vi "Main.vi"() -> ()   [LabVIEW 2016]
doc: "The myRIO Project template acquires acceleration data from the onboard accelerometer and displays the changes of acceleration values in a waveform chart."
panel:
  out "path":bool[][](array[boolean])
  in  "USE MANUAL ROADBLOCKS":bool
  out "raw string data":string
  out "roadblock names":string[](array[string])
  in  "pickupLocations":bool[](array[boolean])=[TRUE, TRUE, FALSE]
  in  "pause":bool
  in  "go":bool
  out "speed":dbl=0.11
  in  "overwrite angle":bool
  in  "Source":u16(ring) items=["Odometry", "Lidar"]
  in  "Max. Speed":dbl=0.11
  out "rotated coordinate system":cluster{"Line":cluster{"X":dbl, "Y":dbl}[]}[](graph)=[{"Line"=[{"X"=28.576616461317627, "Y"=357.36358956169147}, {"X"=-4.74077116119355, "Y"=343.61280769162283}, {"X"=-7.350479867352021, "Y"=344.4851372177861}, {"X"=-8.138056777246447, "Y"=346.20981930296045}, {"X"=-7.0881796754405855, "Y"=348.7533004615932}, {"X"=-8.765481040597024, "Y"=350.0749055793108}, {"X"=-8.600379041051553, "Y"=352.2039244346708}, {"X"=-8.419805687206917, "Y"=354.32624780014754}, {"X"=-8.223837019347911, "Y"=356.44176618363844}, {"X"=-8.938032992413582, "Y"=358.1715820073938}, {"X"=-9.64160157058302, "Y"=359.9057474919626}, {"X"=-11.264578053362584, "Y"=361.2767942037909}, {"X"=-11.949049611130476, "Y"=363.0251766457427}, {"X"=-12.622780410928328, "Y"=364.77772601341337}, {"X"=-13.285745087172302, "Y"=366.53437632430945}, {"X"=-8.305129505171124, "Y"=370.3618672176699}, {"X"=-8.933911813679401, "Y"=372.091919800773}, {"X"=-9.552066882451356, "Y"=373.82579795183943}, {"X"=-8.269612100595452, "Y"=376.2176945222226}, {"X"=-8.862464396842654, "Y"=377.94741894033393}, {"X"=-10.393615033779838, "Y"=379.3652403911355}, {"X"=-10.016273419447543, "Y"=381.41761785287076}, {"X"=-10.577186705547717, "Y"=383.15796169626856}, {"X"=-8.263702090581091, "Y"=385.7956786540522}, {"X"=-8.797785092278218, "Y"=387.52518650617935}, {"X"=-9.321245979333298, "Y"=389.25793887250137}, {"X"=-9.834065043739827, "Y"=390.99387051587115}, {"X"=-13.22100825471199, "Y"=391.9095000800054}, {"X"=-13.717484233486346, "Y"=393.6693102999656}, {"X"=-10.343589355728568, "Y"=396.4827380376795}, {"X"=-10.81205864051907, "Y"=398.22480665727596}, {"X"=-11.269829974406946, "Y"=399.96971695641616}, {"X"=-9.777762208684806, "Y"=402.2070954360229}, {"X"=-9.240072095703283, "Y"=404.18447681452164}, {"X"=-9.661305173161736, "Y"=405.91962939644634}, {"X"=-10.071883624935197, "Y"=407.6573339521877}, {"X"=-10.471791992977046, "Y"=409.39752505815153}, {"X"=-10.861015220963111, "Y"=411.1401371971261}, {"X"=-11.239538654859018, "Y"=412.8851047607493}, {"X"=-14.54489110801353, "Y"=414.0233951038116}, {"X"=-8.042797116220015, "Y"=417.16975136641827}, {"X"=-8.384376585253563, "Y"=418.89731316305176}, {"X"=-8.715349504241715, "Y"=420.6269383310432}, {"X"=-9.035703412241162, "Y"=422.3585617509825}, {"X"=-9.34542624810831, "Y"=424.0921182282268}, {"X"=-9.644506350953407, "Y"=425.8275424953543}, {"X"=-9.93293246057965, "Y"=427.5647692146224}, {"X"=-11.198655470293886, "Y"=429.14903464229513}, {"X"=-11.466672030825464, "Y"=430.89573491513625}, {"X"=-11.723965994630248, "Y"=432.64404682553766}, {"X"=-18.905020724190877, "Y"=433.43849566056014}, {"X"=-14.189269156327327, "Y"=435.8844303075074}, {"X"=-9.454690928780451, "Y"=438.2709538865383}, {"X"=-9.666769274690068, "Y"=440.0067816765684}, {"X"=-9.868192789194438, "Y"=441.7438780783978}, {"X"=-10.058953888811914, "Y"=443.4821776913292}, {"X"=-7.254062500877922, "Y"=445.5214102373096}, {"X"=-7.421694309173745, "Y"=447.24359873735864}, {"X"=-4.590318737091252, "Y"=449.22992564923106}, {"X"=-7.725241095683145, "Y"=450.6908993097107}, {"X"=-9.855438786401749, "Y"=452.2649151077689}, {"X"=-9.981644256507991, "Y"=454.00293840806137}, {"X"=-10.097183040343793, "Y"=455.74170337276314}, {"X"=-10.2020507879393, "Y"=457.48114453835586}, {"X"=-10.296243551082966, "Y"=459.221196415863}, {"X"=-10.379757783470552, "Y"=460.96179349331453}, {"X"=-12.451089774345235, "Y"=462.62541047915863}, {"X"=-12.51367557754827, "Y"=464.3791653611051}, {"X"=-12.565499364932691, "Y"=466.13327124838077}, {"X"=-12.606559185362244, "Y"=467.8876620998903}, {"X"=-11.636954252712883, "Y"=469.6564672629717}, {"X"=-11.656413628399832, "Y"=471.4050943456118}, {"X"=-7.665150667473995, "Y"=473.1615040251902}, {"X"=-6.663187179987403, "Y"=474.8814827168105}, {"X"=-6.650680093319181, "Y"=476.5994929789812}, {"X"=-6.627631729298514, "Y"=478.31739415805316}, {"X"=-6.594042955683392, "Y"=480.03512157601784}, {"X"=-6.5499150370721395, "Y"=481.752610561409}, {"X"=-6.495249634855895, "Y"=483.4697964517369}, {"X"=-6.430048807156254, "Y"=485.1866145959235}, {"X"=-7.3532030238397965, "Y"=486.95014622935224}, {"X"=-7.266631020635884, "Y"=488.67216315996683}, {"X"=-8.167728798156418, "Y"=490.45301669341313}, {"X"=-8.059648252626573, "Y"=492.17996551967616}, {"X"=-5.946113080761734, "Y"=493.7629274424393}, {"X"=-5.817765125964911, "Y"=495.47618238279114}, {"X"=-5.678907252593433, "Y"=497.18861754335745}, {"X"=-4.533602281761773, "Y"=498.8101755503944}, {"X"=-4.374311584895565, "Y"=500.5146684743988}, {"X"=-4.204565314664592, "Y"=502.21815192246373}, {"X"=-9.98907306792114, "Y"=504.57041994725495}, {"X"=-1.8468641884958856, "Y"=505.3930189953423}, {"X"=-9.588938254255936, "Y"=508.0449096021341}, {"X"=-10.364844281303931, "Y"=509.9068374384244}, {"X"=-9.14619623718312, "Y"=511.514227364647}, {"X"=-7.918541104854057, "Y"=513.1080304041075}, {"X"=-8.660913692021893, "Y"=514.9778507683}, {"X"=-7.4137925848477835, "Y"=516.5564685803645}, {"X"=-7.145558462231008, "Y"=518.2782999508851}, {"X"=-7.853387999552297, "Y"=520.1614681851706}, {"X"=-9.534235248411392, "Y"=522.224060739526}, {"X"=-9.231185517333586, "Y"=523.9587962108145}, {"X"=-10.884409037757564, "Y"=526.0539356004363}, {"X"=-10.557834219672543, "Y"=527.7968834860404}, {"X"=-8.258253373376306, "Y"=529.1513889314982}, {"X"=-4.972857724789094, "Y"=530.2805060927069}, {"X"=-9.514030681444524, "Y"=533.0132452292144}, {"X"=-8.16734377467003, "Y"=534.5364235287593}, {"X"=-7.788772537104705, "Y"=536.2625401348871}, {"X"=-7.399617173649688, "Y"=537.9863013779125}, {"X"=-6.9998923357846365, "Y"=539.7076423591985}, {"X"=-6.589613072923612, "Y"=541.4264982712307}, {"X"=-6.16879483184897, "Y"=543.1428044000553}, {"X"=-5.737453456129742, "Y"=544.8564961277164}, {"X"=-6.263070235534087, "Y"=546.8205136322952}, {"X"=-5.809161085484845, "Y"=548.5347145911218}, {"X"=-5.344742340798291, "Y"=550.2460981464135}, {"X"=-2.9445431772094253, "Y"=551.4130604618009}, {"X"=-2.462517159902575, "Y"=553.106812867996}, {"X"=-1.9701075472106027, "Y"=554.797575733741}, {"X"=-14.872292004672545, "Y"=560.5234868358712}, {"X"=-15.289850128660532, "Y"=562.5845676530818}, {"X"=-14.739044634956315, "Y"=564.3538591382237}, {"X"=-14.177393341546122, "Y"=566.1197376379802}, {"X"=-13.604917394283916, "Y"=567.8821366680233}, {"X"=-13.021638346565624, "Y"=569.6409898750259}, {"X"=-12.42757815851752, "Y"=571.3962310391589}, {"X"=-9.934301657009087, "Y"=572.4892136921314}, {"X"=-13.091585246825389, "Y"=575.565768386433}, {"X"=-8.700702889770241, "Y"=575.9579170572881}, {"X"=-9.005971749992511, "Y"=578.0331411139174}, {"X"=-8.360493883773245, "Y"=579.7635846311488}, {"X"=-7.704410366678644, "Y"=581.4900349955396}, {"X"=-7.037745899882566, "Y"=583.2124272072089}, {"X"=-11.006619516480896, "Y"=586.7783465917362}, {"X"=-11.234378317351457, "Y"=588.8961258843899}, {"X"=-10.52220448051105, "Y"=590.6400381546518}, {"X"=-9.79934360561333, "Y"=592.379547779745}, {"X"=-9.06582290796166, "Y"=594.1145892681152}, {"X"=-8.321670004195653, "Y"=595.8450972964314}, {"X"=-7.56691291125162, "Y"=597.571006712044}, {"X"=-7.714074863751819, "Y"=599.7013407976909}, {"X"=-6.02570022071302, "Y"=601.0087699626846}, {"X"=-7.96152054987607, "Y"=603.9812598891432}, {"X"=-7.1568476814880455, "Y"=605.7048063082864}, {"X"=-6.341614478824056, "Y"=607.4233829022542}, {"X"=-5.515851634953492, "Y"=609.1369249676097}, {"X"=-4.679590239380502, "Y"=610.8453679904626}, {"X"=-4.726949489757828, "Y"=612.9965395573656}, {"X"=-11.888924814779273, "Y"=618.7803947764087}, {"X"=-10.993372229540284, "Y"=620.5277607055597}, {"X"=-10.08711486704459, "Y"=622.2695987336806}, {"X"=-10.053013460071043, "Y"=624.4755423042335}, {"X"=-5.60283876818562, "Y"=624.3111076715884}, {"X"=-4.673468700387673, "Y"=626.0197987877557}, {"X"=-8.103788909902335, "Y"=630.1521022214033}, {"X"=-7.138532093630772, "Y"=631.8760289240817}, {"X"=-5.294712387779498, "Y"=633.0974419467224}, {"X"=-5.176376265912438, "Y"=635.3059521780373}, {"X"=-6.765084175222, "Y"=638.5333381993366}, {"X"=-5.748426262510748, "Y"=640.2488929897848}, {"X"=-7.287928028799342, "Y"=643.5113098946317}, {"X"=-7.9454418991443845, "Y"=646.2758804458762}, {"X"=-8.579530684886436, "Y"=649.0548736967197}, {"X"=-11.727686448201723, "Y"=653.4482191933557}, {"X"=-10.61941912656988, "Y"=655.193943170491}, {"X"=-9.500461106804153, "Y"=656.9328340844199}, {"X"=-8.370854517041835, "Y"=658.6648264668819}, {"X"=-3.9004938613651916, "Y"=658.1739773753948}, {"X"=-2.7633771773371905, "Y"=659.8715856406279}, {"X"=-1.615865570714334, "Y"=661.5621847320599}, {"X"=0.36419694891867493, "Y"=662.6765111347985}, {"X"=-3.383286648068747, "Y"=667.7932714052793}, {"X"=-5.447766123981808, "Y"=671.8045116821027}, {"X"=-5.850150506567218, "Y"=674.6798321014182}, {"X"=-4.611719100169125, "Y"=676.3890925168814}, {"X"=-6.580231930976424, "Y"=680.4673331146699}, {"X"=-6.907658127202353, "Y"=683.379118347888}, {"X"=-5.615828996583957, "Y"=685.0947037465218}, {"X"=-9.073174580468503, "Y"=690.4554761805456}, {"X"=-7.737884969217532, "Y"=692.184215727906}, {"X"=-7.177761300675797, "Y"=694.523276104051}, {"X"=-6.599485849851021, "Y"=696.86366520989}, {"X"=-6.78111983557892, "Y"=699.8333904921269}, {"X"=-5.3883315711452155, "Y"=701.5478897193765}, {"X"=-2.444386340660799, "Y"=701.9785237132016}, {"X"=-1.0385174240079778, "Y"=703.6663728624455}, {"X"=-3.434562208301088, "Y"=708.580807116901}, {"X"=-1.9881638024811537, "Y"=710.274607584932}, {"X"=-2.04030174789159, "Y"=713.2722138796564}, {"X"=-3.566781716796527, "Y"=717.601263778914}, {"X"=-3.5577118068576965, "Y"=720.6268360737213}, {"X"=-13.171025825242452, "Y"=732.3731469219651}, {"X"=-12.316573107347551, "Y"=734.8009151196794}, {"X"=-10.709123941989048, "Y"=736.5487209959161}, {"X"=-8.36119953858173, "Y"=737.602950034046}, {"X"=-7.462204307042384, "Y"=740.014579243237}, {"X"=-6.544192478265359, "Y"=742.4250859977826}, {"X"=-5.607144139577372, "Y"=744.8343275597374}, {"X"=-6.78938941218064, "Y"=749.3463147892161}, {"X"=-5.801261365891946, "Y"=751.7656776696217}, {"X"=-3.3857187638355413, "Y"=752.7631082289083}, {"X"=-1.6682237743222572, "Y"=754.4557772798655}, {"X"=-2.721797020952863, "Y"=759.0125399333904}, {"X"=-9.257161622796275, "Y"=769.376046154616}, {"X"=-8.124105020179286, "Y"=771.8315738894411}, {"X"=-6.2895189261544715, "Y"=773.5529581734131}, {"X"=-6.476932476945194, "Y"=777.469596394551}, {"X"=-4.60778313473719, "Y"=779.1807676836203}, {"X"=-9.412491430211844, "Y"=788.3181686710523}, {"X"=-10.796000795056557, "Y"=793.786450495438}, {"X"=-9.48590644158304, "Y"=796.2757356954651}, {"X"=-9.465193730872045, "Y"=800.2728678468713}, {"X"=-7.456069892235803, "Y"=802.0019454971552}, {"X"=-9.953492337332364, "Y"=809.0661525397925}, {"X"=-10.452816880429737, "Y"=813.8695496847113}, {"X"=-14.71904081923617, "Y"=823.3223156412832}, {"X"=-14.461784812557255, "Y"=827.4102231493271}, {"X"=-12.286055232686806, "Y"=829.1694484530829}, {"X"=-10.099572206775065, "Y"=830.9152906141896}, {"X"=-7.90241805467241, "Y"=832.6476839026767}, {"X"=-8.142298346368534, "Y"=837.5302859639576}, {"X"=-10.76092125893905, "Y"=845.6079084090223}, {"X"=-8.473602449144096, "Y"=847.3440830746283}, {"X"=-6.175673730000483, "Y"=849.0661903328643}, {"X"=-3.867221617225141, "Y"=850.7741653473654}, {"X"=-14.4701675724736, "Y"=870.2731731543768}, {"X"=-12.031435717846477, "Y"=872.0316430108596}, {"X"=-10.736720367624855, "Y"=875.4080668442864}, {"X"=-8.266551678719338, "Y"=877.1435320364542}, {"X"=-9.18968465743086, "Y"=883.8048036432882}, {"X"=-6.668023682607554, "Y"=885.5306183365925}, {"X"=-5.807327705133503, "Y"=889.732125342123}, {"X"=-9.874120088076722, "Y"=901.4427014978764}, {"X"=-9.43196911126148, "Y"=906.5210795125762}, {"X"=-6.770919127109551, "Y"=908.247953207868}, {"X"=-7.8556784022915735, "Y"=915.8652250552609}, {"X"=-7.794495750848455, "Y"=921.8177480003112}, {"X"=-8.196978458223043, "Y"=928.6363521433555}, {"X"=-13.736242524766965, "Y"=944.01214617937}, {"X"=-12.90807900096081, "Y"=949.191676137402}, {"X"=-10.49562725444406, "Y"=951.7989619216245}, {"X"=-9.072336663828139, "Y"=956.1205170615633}, {"X"=-10.106116753702281, "Y"=964.7729386898258}, {"X"=-12.033340910816094, "Y"=975.1942226072335}, {"X"=-9.440100589363794, "Y"=977.8079205692866}, {"X"=-6.34164261841255, "Y"=979.5335022037527}, {"X"=-7.539061333916038, "Y"=989.1428785911435}, {"X"=-5.317274566394929, "Y"=992.6186075930843}, {"X"=-4.466407579703116, "Y"=998.7381077790387}, {"X"=-3.0886008324087584, "Y"=1003.9797849534243}, {"X"=-9.422390748874534, "Y"=1024.34690294733}, {"X"=-7.3923625430387006, "Y"=1028.7485725817364}, {"X"=-7.993983839324244, "Y"=1038.5166213778946}, {"X"=-4.963396007688061, "Y"=1041.130015874826}, {"X"=-9.73820276004102, "Y"=1059.936700929226}, {"X"=-6.994393661101242, "Y"=1063.4688956165824}, {"X"=-4.217863479354435, "Y"=1066.9894223036495}, {"X"=-8.099501387073303, "Y"=1085.03185348001}, {"X"=-5.580944645459169, "Y"=1089.479932503771}, {"X"=-3.0183513268182196, "Y"=1093.920017711641}, {"X"=-4.826984283811328, "Y"=1108.4267291040496}, {"X"=-2.1144303473452055, "Y"=1112.8766086225169}, {"X"=-7.5501607217547075, "Y"=1136.653061681427}, {"X"=-3.4770828654445154, "Y"=1138.3640566479803}, {"X"=-2.802682121336943, "Y"=1148.3793758627119}, {"X"=-5.373595942088059, "Y"=1166.7612389698077}, {"X"=-5.892059617806865, "Y"=1180.5491152580664}, {"X"=-2.6347402787606597, "Y"=1185.046005847571}, {"X"=-3.6042542742794126, "Y"=1200.74343475171}, {"X"=-5.4419866034307915, "Y"=1219.2890159791455}, {"X"=-7.062321077849106, "Y"=1237.8838873573395}, {"X"=-4.739017247575703, "Y"=1246.1762423118103}, {"X"=-1.3256554817880328, "Y"=1251.6397452980111}, {"X"=-3.0897310820254233, "Y"=1272.2099762036185}, {"X"=-2.362195675266321, "Y"=1286.201649046942}, {"X"=-3.3662561011780667, "Y"=1305.9075309674656}, {"X"=-2.2805666636053274, "Y"=1319.9506001401144}, {"X"=-0.42513081455462043, "Y"=1332.105766246754}, {"X"=2.1651956347232613, "Y"=1342.3604898886258}, {"X"=-2.724098560849768, "Y"=1377.4813018627735}, {"X"=1.109073246825858, "Y"=1384.907078098183}, {"X"=-1.1450318426243484, "Y"=1413.4372678254877}, {"X"=-0.8631985957002826, "Y"=1434.3356531193622}, {"X"=0.7392338813229458, "Y"=1451.4121917703867}, {"X"=2.2784130196424144, "Y"=1469.469543667663}, {"X"=1.9752874456671066, "Y"=1495.2760742742785}, {"X"=1.72809958998522, "Y"=1522.0909465154327}, {"X"=2.0448527388076627, "Y"=1547.9768043111544}, {"X"=2.669275799484467, "Y"=1573.8973336442273}, {"X"=1.2725041271489772, "Y"=1609.5746679412048}, {"X"=1.665421931336084, "Y"=1639.4658562714153}, {"X"=1.9732061027862642, "Y"=1671.3444819554675}, {"X"=3.522186165777555, "Y"=1699.3556174324276}, {"X"=4.7779344628372655, "Y"=1730.325593190843}, {"X"=4.982894058226975, "Y"=1768.1794664657875}, {"X"=7.612329623712583, "Y"=1796.272690601469}, {"X"=7.330335818030846, "Y"=1841.068557357675}, {"X"=7.03358539097519, "Y"=1888.864307100026}, {"X"=8.029275882144532, "Y"=1932.7779692274896}, {"X"=6.4426973114146335, "Y"=1994.4601436141454}, {"X"=10.107360058679774, "Y"=2029.5927571615584}, {"X"=13.228782674090837, "Y"=2070.6583560051076}, {"X"=-9.24412840866512, "Y"=2977.808666395851}, {"X"=6.126099747780017, "Y"=2979.4953961187844}]}, {"Line"=[{"X"=68.62973356513766, "Y"=4051.851402285283}, {"X"=90.94562316458712, "Y"=4046.0491940237675}, {"X"=112.9134263637961, "Y"=4046.102068397886}, {"X"=135.1073891816279, "Y"=4040.0243951170473}, {"X"=156.99253314549912, "Y"=4040.8054046682064}, {"X"=178.88205731223576, "Y"=4041.4521147981895}, {"X"=200.75480715528755, "Y"=4042.964294474817}, {"X"=222.58577721259627, "Y"=4048.341939900227}, {"X"=244.52030991588802, "Y"=4048.586035577704}, {"X"=266.45592745072076, "Y"=4048.6955388976476}, {"X"=288.3918039534931, "Y"=4048.670445737322}, {"X"=310.32711355085127, "Y"=4048.5107570414684}, {"X"=332.2610303907877, "Y"=4048.2164788222763}, {"X"=354.19272867373047, "Y"=4047.7876221591546}, {"X"=376.1213826836351, "Y"=4047.2242031983146}, {"X"=398.1508201093675, "Y"=4049.524417211289}, {"X"=420.17133524166366, "Y"=4050.689560763215}, {"X"=442.11655318347863, "Y"=4049.7212500549867}, {"X"=464.10869061670405, "Y"=4049.616884178716}, {"X"=486.0464996304325, "Y"=4048.3789991189515}, {"X"=507.97630015117113, "Y"=4047.006529496461}, {"X"=530.2554945953639, "Y"=4050.4866777392676}, {"X"=552.5084528865657, "Y"=4052.8307942088063}, {"X"=574.4643179809686, "Y"=4051.0504379037943}, {"X"=596.4088457014934, "Y"=4049.135396457895}, {"X"=618.3412098490757, "Y"=4047.0857419713357}, {"X"=640.2605846826016, "Y"=4044.9015516124505}, {"X"=662.4910740439232, "Y"=4045.565259217772}, {"X"=684.4002882619448, "Y"=4043.1101990075686}, {"X"=706.7760296379319, "Y"=4044.4916054787773}, {"X"=728.6778223886847, "Y"=4041.7648381005847}, {"X"=752.5525807322003, "Y"=4053.771131255632}, {"X"=776.3142398765136, "Y"=4063.637560662127}, {"X"=798.4770279617144, "Y"=4061.47321142267}, {"X"=821.6884553762941, "Y"=4066.091855419856}, {"X"=844.8193293479787, "Y"=4069.572828702131}, {"X"=867.3614643563512, "Y"=4068.958442120934}, {"X"=890.9319526498374, "Y"=4074.116323245808}, {"X"=913.0120525683635, "Y"=4070.259038689616}, {"X"=935.2492170083682, "Y"=4067.2498016412865}, {"X"=958.9709613722258, "Y"=4071.9616531487213}, {"X"=981.2297625705849, "Y"=4068.6680884687785}, {"X"=1004.470050173194, "Y"=4070.1365788299113}, {"X"=1028.986337704895, "Y"=4077.3272810986987}, {"X"=1051.5060010466395, "Y"=4074.5777230442354}, {"X"=1074.454803523784, "Y"=4073.639653488076}, {"X"=1097.6445680760262, "Y"=4073.530156097562}]}, {"Line"=[{"X"=1119.7171800339775, "Y"=4068.404517812021}, {"X"=1140.5821563252948, "Y"=4058.283750349535}, {"X"=1158.2203692848036, "Y"=4035.4259937316024}, {"X"=1180.0580381754864, "Y"=4029.929386617402}, {"X"=1050.5647602626423, "Y"=3445.754789652453}, {"X"=1051.9554489777408, "Y"=3378.146707373487}, {"X"=1030.828012502977, "Y"=3231.564248258306}, {"X"=1036.092579394132, "Y"=3185.470739769273}, {"X"=1034.733686827593, "Y"=3118.276794454778}, {"X"=1050.9461586273483, "Y"=3113.5551524543307}, {"X"=1059.9182797935512, "Y"=3084.796694468842}, {"X"=1075.9248474689043, "Y"=3079.9211529644413}, {"X"=1091.3280021602448, "Y"=2965.893029738508}, {"X"=1013.5246698545084, "Y"=2683.004819677823}, {"X"=1013.4801690657687, "Y"=2638.679785413157}, {"X"=1015.5544224957287, "Y"=2601.99380265851}, {"X"=1012.1805965157625, "Y"=2551.2322263959277}, {"X"=1016.733711927881, "Y"=2524.0968394413107}, {"X"=1018.5556512867352, "Y"=2490.4185915035937}, {"X"=1013.650148164828, "Y"=2439.9507385324455}, {"X"=1014.9579084520163, "Y"=2407.3607263831773}, {"X"=1018.4407590605125, "Y"=2381.350029245549}, {"X"=1016.8287587005875, "Y"=2343.290354886976}, {"X"=1017.7800497470034, "Y"=2312.739015139495}, {"X"=1019.5275249617839, "Y"=2285.021209814635}, {"X"=1020.9632401463714, "Y"=2257.3520688553735}, {"X"=1016.5967428890236, "Y"=2216.856189499879}, {"X"=1019.3213483880911, "Y"=2193.9138776527684}, {"X"=1018.5648413360177, "Y"=2163.6845475913196}, {"X"=1019.9204078264515, "Y"=2139.0051996852203}, {"X"=1022.6602295001629, "Y"=2118.0134693602495}, {"X"=1019.7075178112838, "Y"=2085.2551533989995}, {"X"=1017.2331358182465, "Y"=2054.405659385074}, {"X"=1016.5655353814343, "Y"=2028.1590946955357}, {"X"=1020.4099901631861, "Y"=2011.8757342727413}, {"X"=1017.4468534987415, "Y"=1982.1518738494772}, {"X"=1016.8348972721142, "Y"=1957.8877594114003}, {"X"=1015.9535638301378, "Y"=1933.6886875999896}, {"X"=1015.2624628727638, "Y"=1910.4455723968601}, {"X"=1012.4573566969317, "Y"=1883.723840342923}, {"X"=1015.4587850504512, "Y"=1868.5682040926208}, {"X"=1006.424589128683, "Y"=1831.431021012615}, {"X"=1010.4171809500516, "Y"=1819.0143390067162}, {"X"=1011.3699449736303, "Y"=1801.3558871886341}, {"X"=1009.6779176549045, "Y"=1779.3817184615168}, {"X"=1015.1927627632011, "Y"=1770.4990038675662}, {"X"=1014.6039159228995, "Y"=1751.218652913763}, {"X"=1016.3425811759449, "Y"=1736.3041271619893}, {"X"=1006.1399718658224, "Y"=1701.6662801345756}, {"X"=1010.0368473807367, "Y"=1691.1578635270755}, {"X"=1009.648886749731, "Y"=1673.829179453594}, {"X"=1013.3016709618233, "Y"=1663.344679285377}, {"X"=1013.1200550796127, "Y"=1646.9395914182674}, {"X"=1010.6110550429743, "Y"=1627.211596625122}, {"X"=1014.9564208318981, "Y"=1618.4696753174699}, {"X"=1012.0873096797006, "Y"=1598.8510501078233}, {"X"=1015.0994006564265, "Y"=1588.4692073818312}, {"X"=1009.066969983661, "Y"=1564.8270257392296}, {"X"=1012.363270980889, "Y"=1555.3380574418038}, {"X"=1018.4169522286022, "Y"=1549.9609004190033}, {"X"=1016.3932147294128, "Y"=1533.0885315554222}, {"X"=1015.9285396073809, "Y"=1518.7274373905484}, {"X"=1016.4843407585715, "Y"=1506.0354647699226}, {"X"=1018.0909795856861, "Y"=1494.992287050514}, {"X"=1024.3434781895098, "Y"=1490.4033206540628}, {"X"=1028.7704706177142, "Y"=1483.3740018561687}, {"X"=1027.0997565242478, "Y"=1468.3587201690593}, {"X"=1024.0558004328807, "Y"=1451.8157857501121}, {"X"=1029.429547068251, "Y"=1446.4015039948904}, {"X"=1022.3942071351466, "Y"=1425.2431689571097}, {"X"=1022.6084466507377, "Y"=1413.5916691820128}, {"X"=1027.733253094943, "Y"=1408.1984180027807}, {"X"=1020.1620118847411, "Y"=1387.2930997190624}, {"X"=1015.5513459490553, "Y"=1370.3681473908323}, {"X"=1019.7544967201261, "Y"=1364.2643007085246}, {"X"=1020.6754917849005, "Y"=1354.3304469232596}, {"X"=1020.199424227129, "Y"=1342.902092664586}, {"X"=1020.9241809908161, "Y"=1333.0218948437764}, {"X"=1014.946250357561, "Y"=1315.6616315468327}, {"X"=1014.7739345411102, "Y"=1305.1246188293428}, {"X"=1011.8199042673019, "Y"=1291.6526774145625}, {"X"=1012.7768097563412, "Y"=1282.6773212635092}, {"X"=1015.689097987453, "Y"=1275.9230715355757}, {"X"=1019.913777555941, "Y"=1270.623185561046}, {"X"=1024.7895389205341, "Y"=1266.0272583714393}, {"X"=1019.2482353552157, "Y"=1250.5814546477213}, {"X"=1017.0310567966851, "Y"=1238.8192564653107}, {"X"=1014.6978809083519, "Y"=1227.1137860271683}, {"X"=1014.3665569524621, "Y"=1217.5914202682566}, {"X"=1013.9464746358027, "Y"=1208.1016726759365}, {"X"=1012.7236371042584, "Y"=1197.945520772644}, {"X"=1012.8415963269144, "Y"=1189.2229467017128}, {"X"=1016.4951093004919, "Y"=1183.9810131963982}, {"X"=1018.6578738802992, "Y"=1177.3482416174363}, {"X"=1012.7225267119625, "Y"=1163.2136449823597}, {"X"=1011.7907702143671, "Y"=1153.9213006751359}, {"X"=1007.8143809794315, "Y"=1141.9745956498396}, {"X"=1011.157224124231, "Y"=1136.7868985351877}, {"X"=1012.9683648061023, "Y"=1130.2556522439131}, {"X"=1016.9829779232074, "Y"=1125.704983684927}, {"X"=1012.6541351490703, "Y"=1113.9288538092244}, {"X"=1015.808621613202, "Y"=1108.7304428988175}, {"X"=1019.691105061685, "Y"=1104.162752057672}, {"X"=1015.0988941744199, "Y"=1092.5246913068793}, {"X"=1018.8819543609001, "Y"=1087.961660340124}, {"X"=1022.6369451006786, "Y"=1083.3755028502126}, {"X"=1026.3637250204772, "Y"=1078.7663915033816}, {"X"=1030.0621538091377, "Y"=1074.1344998300688}, {"X"=1019.5631898066492, "Y"=1058.3785516681746}, {"X"=1023.1366491799887, "Y"=1053.7887710898099}, {"X"=1023.5031972754566, "Y"=1046.7489860442702}, {"X"=1027.005224806081, "Y"=1042.1352489578464}, {"X"=1026.4685775416178, "Y"=1034.5138927065484}, {"X"=1022.6440913337282, "Y"=1024.5513916565376}, {"X"=1025.2006045517392, "Y"=1019.3559876926174}, {"X"=1016.340760045356, "Y"=1005.9966644947135}, {"X"=1018.7763954341275, "Y"=1000.8502622657938}, {"X"=1021.1768798740396, "Y"=995.6940328067155}, {"X"=1024.3656838930979, "Y"=991.0955308305904}, {"X"=1024.218352871098, "Y"=984.2285344036068}, {"X"=1024.8455512385744, "Y"=977.9400792070971}, {"X"=1026.2577455187934, "Y"=972.2152743918103}, {"X"=1021.7678255394345, "Y"=962.6636080659109}, {"X"=1024.7539475579856, "Y"=958.06210190376}, {"X"=1026.8679564017875, "Y"=952.9057377114625}, {"X"=1030.6412086626246, "Y"=948.8045558755323}, {"X"=1025.0386831785436, "Y"=938.8865971176466}, {"X"=1026.17173632581, "Y"=933.2234705003063}, {"X"=1022.9799690352821, "Y"=924.9852320436789}, {"X"=1023.155219041908, "Y"=918.8455409939733}, {"X"=1024.1464474685226, "Y"=913.2259472879117}, {"X"=1025.9630948898828, "Y"=908.1108818595344}, {"X"=1026.8761346374285, "Y"=902.4955182441483}, {"X"=1029.492976034798, "Y"=897.8638007339073}, {"X"=1031.2062077491628, "Y"=892.7322453140972}, {"X"=1033.7630613176327, "Y"=888.0741427655739}, {"X"=1025.7191333594888, "Y"=877.7233268749824}, {"X"=1028.183997228332, "Y"=873.0991749206238}, {"X"=1030.6204414338179, "Y"=868.459985894244}, {"X"=1025.022230913521, "Y"=859.69477051734}, {"X"=1027.376486759155, "Y"=855.0752340584802}, {"X"=1029.702353343744, "Y"=850.441339118785}, {"X"=1031.1019142075568, "Y"=845.3529156598422}, {"X"=1020.7608611237232, "Y"=834.6087636141093}, {"X"=1020.251777368617, "Y"=828.7279658561697}, {"X"=1022.4161142753367, "Y"=824.1382832913321}, {"X"=1021.8271534424024, "Y"=818.2808728412011}, {"X"=1026.66010014705, "Y"=814.9195102909744}, {"X"=1025.999304225189, "Y"=809.0697683484877}, {"X"=1021.6315531799838, "Y"=801.6354794444695}, {"X"=1019.9562113470897, "Y"=795.4548018947403}, {"X"=1021.9163935217769, "Y"=790.8675592468253}, {"X"=1023.848392004843, "Y"=786.2683755007417}, {"X"=1025.7521340576382, "Y"=781.657423813158}, {"X"=1029.4831278793663, "Y"=777.7810837413872}, {"X"=1031.3346868166316, "Y"=773.1357177353177}, {"X"=1031.293110221613, "Y"=767.7556992747046}, {"X"=1029.3451190507744, "Y"=761.6755673924848}, {"X"=1026.4145244480292, "Y"=755.2802438630265}, {"X"=1027.1892803971427, "Y"=750.3096623962425}, {"X"=1026.9905327693778, "Y"=745.0014867406476}, {"X"=1031.4698707639948, "Y"=741.3707956580233}, {"X"=1030.2630439671104, "Y"=735.7325374438414}, {"X"=1027.1217376624934, "Y"=729.4765544091891}, {"X"=1029.6258729227193, "Y"=725.162095019256}, {"X"=1030.2037241792505, "Y"=720.207164025366}, {"X"=1030.749279413522, "Y"=715.2546207580086}, {"X"=1030.3080201561504, "Y"=710.0066867174093}, {"X"=1031.7437076827464, "Y"=705.3575351013521}, {"X"=1028.360069063941, "Y"=699.26840387338}, {"X"=1024.9304400857986, "Y"=693.2295714580689}, {"X"=1026.2632863998426, "Y"=688.6137318774685}, {"X"=1027.567785364206, "Y"=683.9898009975062}, {"X"=1031.7385605037387, "Y"=680.1459061513254}, {"X"=1029.1250615459658, "Y"=674.4616363129907}, {"X"=1030.3426710122935, "Y"=669.8204123200392}, {"X"=1031.5317795424155, "Y"=665.1718045855847}, {"X"=1032.6923423670676, "Y"=660.5159881270813}, {"X"=1025.0718734909847, "Y"=653.7567714304674}, {"X"=1026.1625165948365, "Y"=649.1408070951128}, {"X"=1027.2248161429338, "Y"=644.518237593704}, {"X"=1028.2587321402991, "Y"=639.8892369633695}, {"X"=1029.264225660579, "Y"=635.253979483367}, {"X"=1030.2412588475113, "Y"=630.612639668521}, {"X"=1035.111427339113, "Y"=626.7533003415052}, {"X"=1028.1834050430157, "Y"=620.5485816694733}, {"X"=1029.0702279513848, "Y"=615.9141504702209}, {"X"=1028.9447301208002, "Y"=611.0954675287348}, {"X"=1026.8186948300342, "Y"=605.9379710551757}, {"X"=1025.6439164590947, "Y"=600.978567600785}, {"X"=1026.4107078237107, "Y"=596.3600868105357}, {"X"=1021.2213757739917, "Y"=590.8087979897297}, {"X"=1021.9258498584444, "Y"=586.2176448420196}, {"X"=1022.6021398952505, "Y"=581.6222555497494}, {"X"=1023.2502204224729, "Y"=577.0228031267286}, {"X"=1023.8700670402453, "Y"=572.4194607397415}, {"X"=1024.4616564116932, "Y"=567.8124017020273}, {"X"=1025.0249662638112, "Y"=563.2017994667543}, {"X"=1025.5599753883016, "Y"=558.5878276204915}, {"X"=1028.0553884360988, "Y"=554.1827299000586}, {"X"=1028.5350005432442, "Y"=549.5503335143442}, {"X"=1028.986179771956, "Y"=544.9150814876165}, {"X"=1029.4089091355895, "Y"=540.2771483344952}, {"X"=1024.8198470038583, "Y"=535.2287076649658}, {"X"=1025.1832203250847, "Y"=530.6165209923689}, {"X"=1020.5303296810426, "Y"=525.6553743145482}, {"X"=1020.8350428820744, "Y"=521.0696878407397}, {"X"=1021.1116131037259, "Y"=516.4822180061308}, {"X"=1021.3600299332843, "Y"=511.8931375263673}, {"X"=1025.5762570743432, "Y"=507.48206090352295}, {"X"=1031.7648642329552, "Y"=503.09813458593834}, {"X"=1025.934146036672, "Y"=498.24835172098807}, {"X"=1027.070240933464, "Y"=493.6564886148944}, {"X"=1027.1784895509604, "Y"=489.0312763700058}, {"X"=1027.2583563618941, "Y"=484.4054869923997}, {"X"=1027.3098383593258, "Y"=479.77929464043285}, {"X"=1027.332933604987, "Y"=475.15287348763195}, {"X"=1025.327658969375, "Y"=470.5348214782281}, {"X"=1024.2941220462144, "Y"=465.9310844060941}, {"X"=1024.2323030412877, "Y"=461.32342802936915}, {"X"=1024.1422131520558, "Y"=456.71623770475605}, {"X"=1024.023855770352, "Y"=452.10968689036855}, {"X"=1023.8772353522647, "Y"=447.50394902023845}, {"X"=1024.7015159109142, "Y"=442.85818157432493}, {"X"=1024.498116566616, "Y"=438.2484598167148}, {"X"=1023.2678564006121, "Y"=433.6933469174743}, {"X"=1023.0082496762661, "Y"=429.09259445466796}, {"X"=1022.7204181525323, "Y"=424.4935215166413}, {"X"=1018.4146520618494, "Y"=420.1828837047227}, {"X"=1018.0722380538735, "Y"=415.6121642745697}, {"X"=1017.7017850845575, "Y"=411.04363189977346}, {"X"=1017.3033071012463, "Y"=406.47745858299515}, {"X"=1019.8629335236369, "Y"=401.62550965259487}, {"X"=1029.3542569739766, "Y"=396.0241743657424}, {"X"=1028.863401977253, "Y"=391.3867855626173}, {"X"=1028.3441017379675, "Y"=386.7524958866652}, {"X"=1026.8036625882814, "Y"=382.2419807060197}, {"X"=1021.2685138948066, "Y"=378.2534504775065}, {"X"=1020.6687719980014, "Y"=373.666009390073}, {"X"=1024.9925284227008, "Y"=368.388569213006}, {"X"=1019.38490168554, "Y"=364.5025987011106}, {"X"=1018.7008216068749, "Y"=359.9269740968156}, {"X"=1024.9019155692074, "Y"=354.25692529097205}, {"X"=1021.1949946565736, "Y"=350.13668718895474}, {"X"=1020.4227329275013, "Y"=345.55022649720894}, {"X"=1022.5759902377677, "Y"=340.44325991952053}, {"X"=1021.7442247602639, "Y"=335.8485080742172}, {"X"=1020.8842820731955, "Y"=331.2589463408433}, {"X"=1019.9961945529194, "Y"=326.67474751380547}, {"X"=1019.0799956354282, "Y"=322.09608418559776}, {"X"=1018.1357198150935, "Y"=317.5231287403061}, {"X"=1017.1634026433663, "Y"=312.95605334711956}, {"X"=1018.1153244896207, "Y"=307.96058284196477}, {"X"=1019.0338743176255, "Y"=302.94739492829854}, {"X"=1018.9454879307717, "Y"=298.14589723031685}, {"X"=1014.9383846591686, "Y"=294.2796798626933}, {"X"=1021.5874842232377, "Y"=287.8037536012339}, {"X"=1026.2467428876823, "Y"=281.73367595315136}, {"X"=1026.9896031742978, "Y"=276.6114965891268}, {"X"=1025.7660902750304, "Y"=271.99086493886466}, {"X"=1024.514248745235, "Y"=267.3778276047042}, {"X"=1023.2341257160381, "Y"=262.77255826489306}, {"X"=1021.925769383348, "Y"=258.1752303052204}, {"X"=1024.4262246403873, "Y"=252.45576706043505}, {"X"=1024.012040306463, "Y"=247.5628757704431}, {"X"=1022.6103444724147, "Y"=242.96106093455202}, {"X"=1021.1804388198841, "Y"=238.3679333704743}, {"X"=1019.7223771840116, "Y"=233.78366600686874}, {"X"=1018.2362144599932, "Y"=229.2084314388099}, {"X"=1016.7220066010156, "Y"=224.6424019212926}, {"X"=1015.1798106161491, "Y"=220.0857493627488}, {"X"=1018.3308284161029, "Y"=213.89219435743854}, {"X"=1018.607021128264, "Y"=208.6557172789465}, {"X"=1019.7870475267127, "Y"=203.0652418231909}, {"X"=1019.9884141667168, "Y"=197.79695957421427}, {"X"=1018.2814361550535, "Y"=193.2207700734951}, {"X"=1017.4800948260723, "Y"=188.29704127274402}, {"X"=1018.5092796942266, "Y"=182.64495686659882}, {"X"=1018.5677961594567, "Y"=177.33906832748409}, {"X"=1016.7353176296713, "Y"=172.77198068901004}, {"X"=1023.1963775193543, "Y"=164.78807651987495}, {"X"=1021.286800419869, "Y"=160.1928247089611}, {"X"=1019.3490633325872, "Y"=155.60937634717516}, {"X"=1017.3832392122148, "Y"=151.03790399875663}, {"X"=1021.7943163865506, "Y"=143.65420858873404}, {"X"=1021.5800803415424, "Y"=138.24978097779024}]}]
  in  "split theshold":dbl=100.0
  in  "merge threshold":dbl=40.0
  in  "min line size":i32=30
  in  "max angle deviation":dbl=30.0
  in  "point merge threshold":dbl=250.0
  in  "landmarks":cluster{dbl, dbl}[](array[cluster])=[{0.0, 0.0}, {1045.0, 0.0}, {0.0, 4000.0}, {1045.0, 4000.0}, {6000.0, 0.0}, {6000.0, 4000.0}, {5035.0, 0.0}, {5035.0, 4000.0}]
  out "robotPos":cluster{"xPos":dbl, "yPos":dbl, "Theta":dbl}={"xPos"=261.42426804429823, "yPos"=344.24888089040223, "Theta"=-174.74342712177267}
  in  "stop":bool=TRUE
  out "lidarRobotPos":cluster{"xPos":dbl, "yPos":dbl, "Theta":dbl}={"xPos"=271.14198739770694, "yPos"=290.6045315655434, "Theta"=-176.0086762787874}
  in  "initialPos":cluster{"xPos":dbl, "yPos":dbl, "Theta":dbl}={"xPos"=250.0, "yPos"=250.0, "Theta"=0.0}
  out "nextPoint":cluster{"y":dbl, "x":dbl, "stop?":bool}={"y"=250.0, "x"=250.0, "stop?"=FALSE}
  in  "manualRoadblocks":bool[][](array[boolean])=[[FALSE, TRUE, FALSE, FALSE, FALSE, FALSE, FALSE], [FALSE, TRUE, TRUE, TRUE, TRUE, TRUE, FALSE], [FALSE, FALSE, FALSE, FALSE, FALSE, FALSE, FALSE], [FALSE, TRUE, FALSE, TRUE, FALSE, TRUE, FALSE], [FALSE, FALSE, FALSE, TRUE, FALSE, FALSE, FALSE]]
  out "Field Map":cluster{"Array":dbl[], "Array 2":dbl[]}[](graph)=[{"Array"=[0.0, 6.0, 6.0, 0.0, 1.0, 1.69, 1.0, 4.99, 4.99, 4.99, 1.0, 1.0, 4.99, 4.39, 4.99], "Array 2"=[0.0, 0.0, 4.0, 4.0, 3.4, 1.2, 1.2, 3.4, 4.0, 0.0, 0.0, 4.0, 1.2, 1.2, 1.0]}, {"Array"=[0.0, 0.0, 6000.0, 6000.0, 0.0], "Array 2"=[0.0, 4000.0, 4000.0, 0.0, 0.0]}, {"Array"=[1000.0, 1000.0, 1090.0, 1090.0, 1000.0], "Array 2"=[0.0, 3400.0, 3400.0, 0.0, 0.0]}, {"Array"=[4990.0, 4990.0, 5080.0, 5080.0, 4990.0], "Array 2"=[1000.0, 3400.0, 3400.0, 1000.0, 1000.0]}, {"Array"=[1690.0, 4390.0, 4390.0, 1690.0, 1690.0], "Array 2"=[1000.0, 1000.0, 1200.0, 1200.0, 1000.0]}, {"Array"=[1690.0, 1690.0, 2190.0, 2190.0, 1690.0], "Array 2"=[2900.0, 3400.0, 3400.0, 2900.0, 2900.0]}, {"Array"=[2790.0, 2790.0, 3290.0, 3290.0, 2790.0], "Array 2"=[2900.0, 3400.0, 3400.0, 2900.0, 2900.0]}, {"Array"=[3890.0, 3890.0, 4390.0, 4390.0, 3890.0], "Array 2"=[2900.0, 3400.0, 3400.0, 2900.0, 2900.0]}, {"Array"=[1690.0, 1690.0, 2190.0, 2190.0, 1690.0], "Array 2"=[1800.0, 2300.0, 2300.0, 1800.0, 1800.0]}, {"Array"=[2790.0, 2790.0, 3290.0, 3290.0, 2790.0], "Array 2"=[1800.0, 2300.0, 2300.0, 1800.0, 1800.0]}, {"Array"=[3890.0, 3890.0, 4390.0, 4390.0, 3890.0], "Array 2"=[1800.0, 2300.0, 2300.0, 1800.0, 1800.0]}, {"Array"=array[8924 elements], "Array 2"=array[8924 elements]}, {"Array"=[250.0], "Array 2"=[250.0]}, {"Array"=array[8924 elements], "Array 2"=array[8924 elements]}]
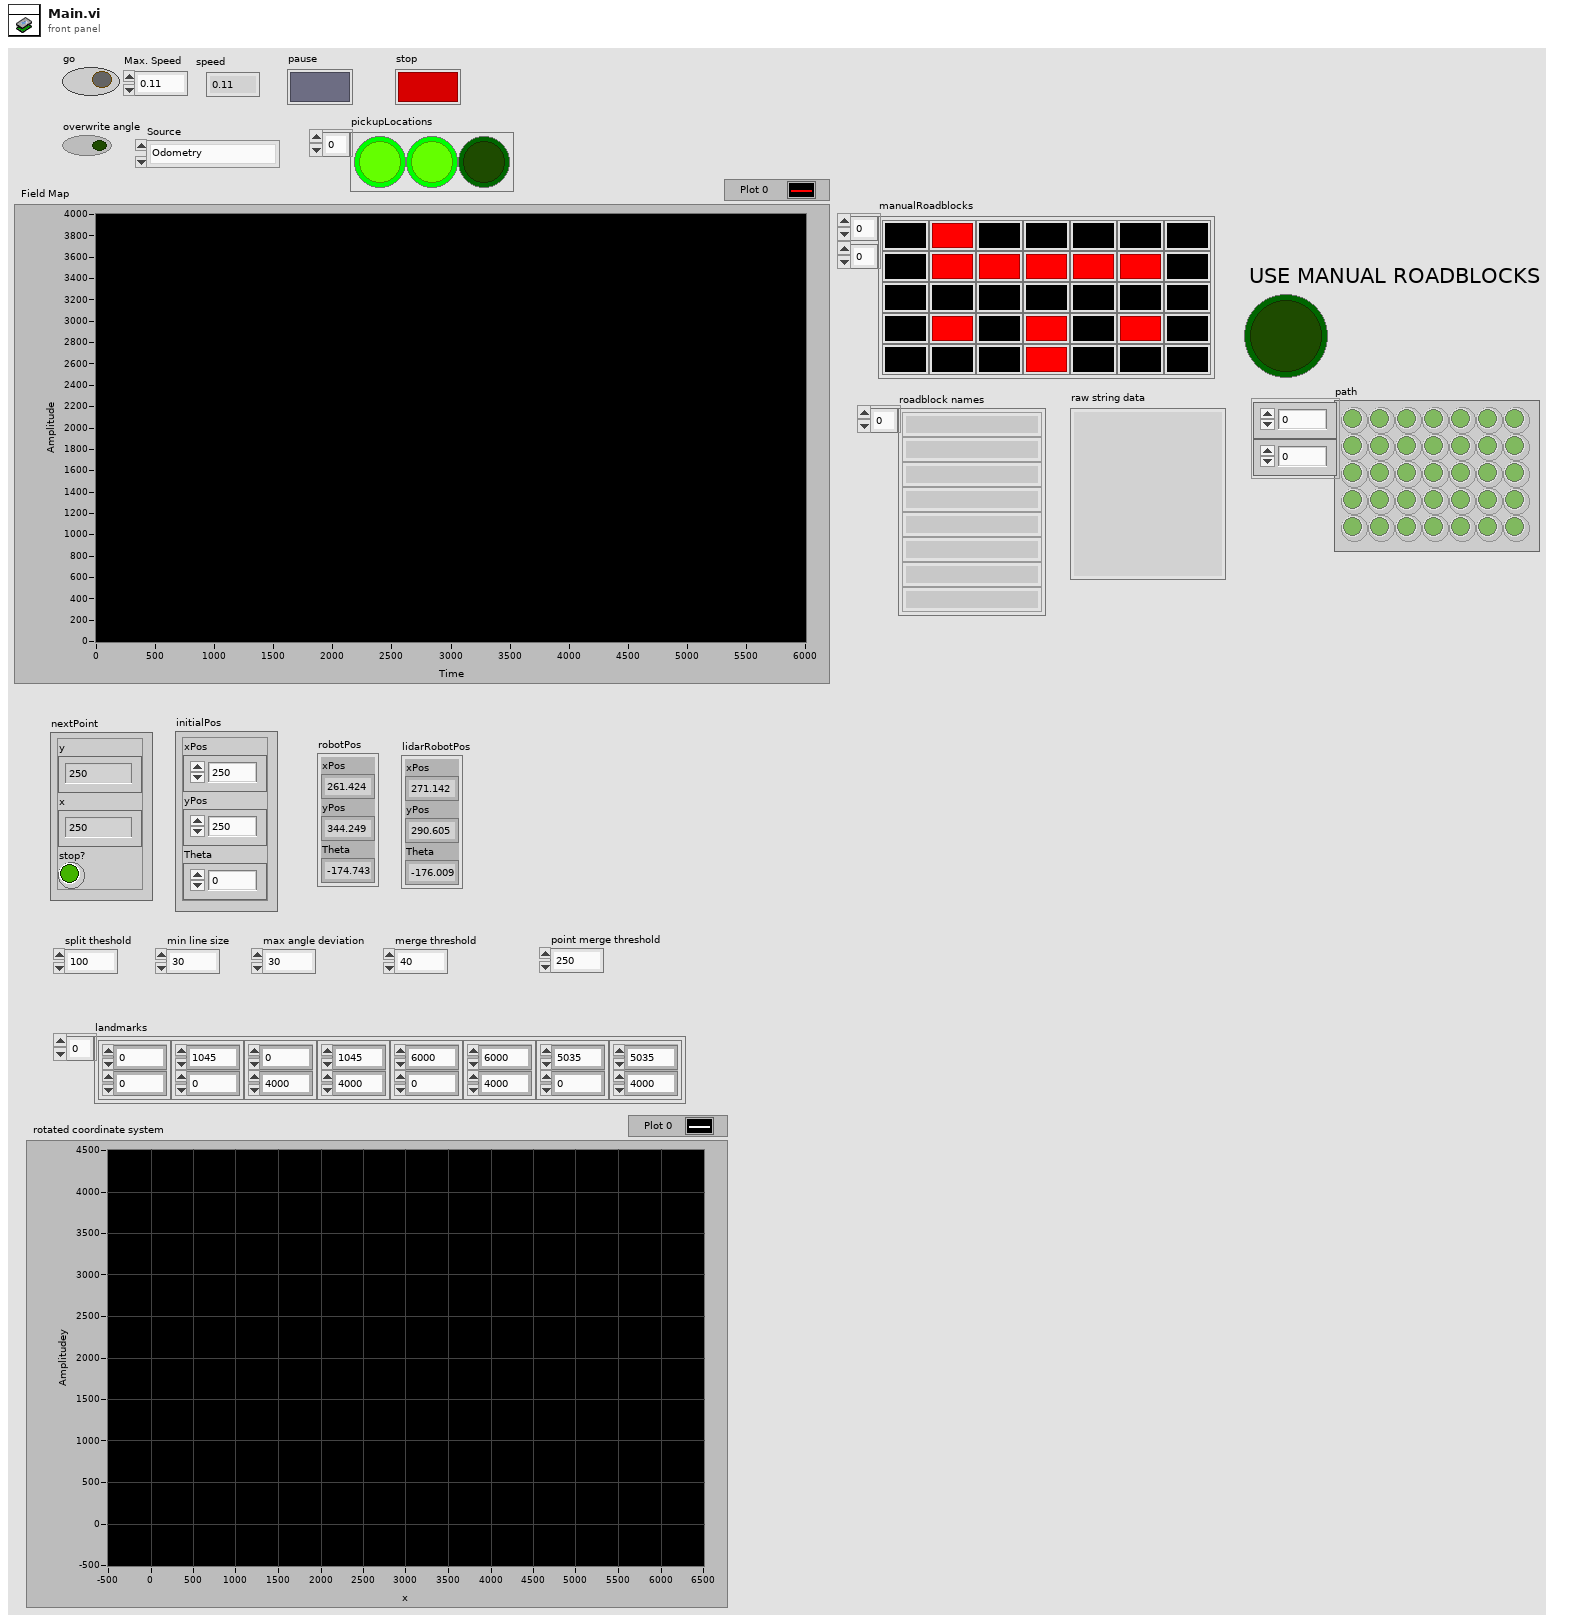
[diagram p1: front panel]
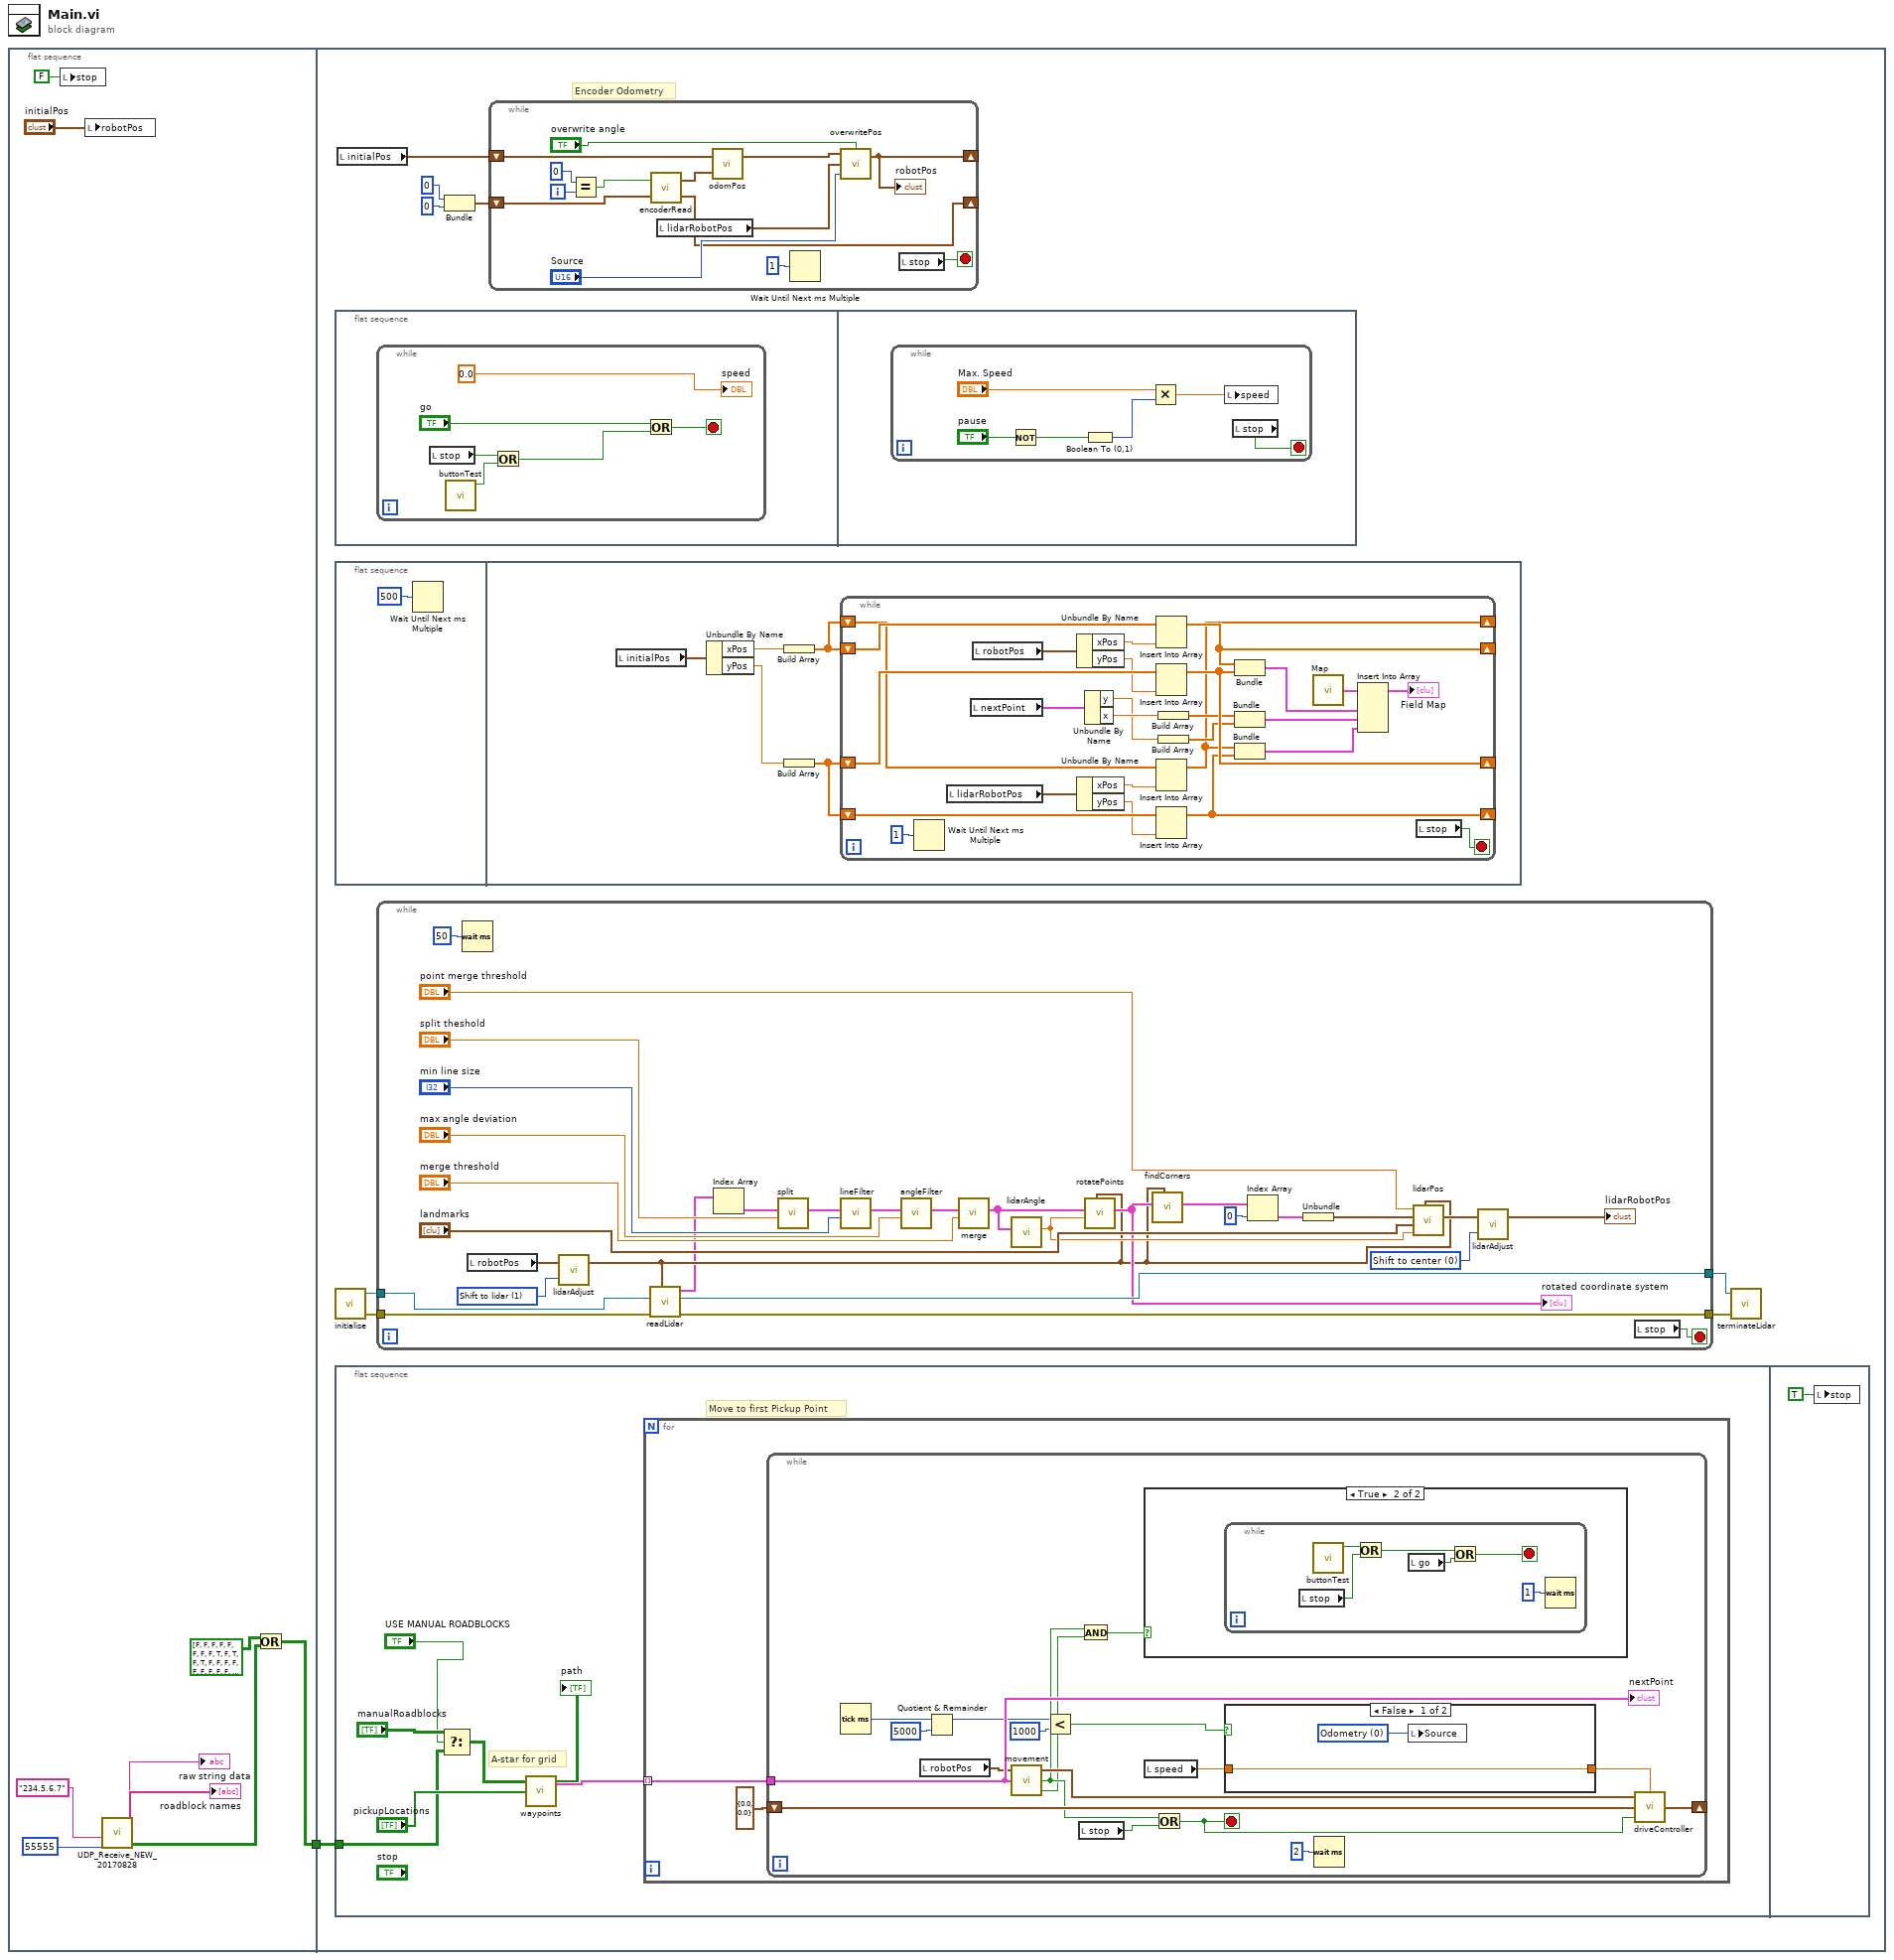
[diagram p0: block diagram]
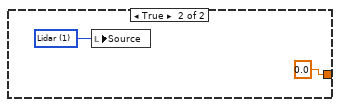
[diagram p2: hidden frame]
diagram:
  n1 = flat-sequence {
    tunnel: [w2] -> w1
    tunnel: w1 -> [w11]
    frame #0 {
      n2 = local write "stop"(FALSE ("stop")) -> ()
      n3 = local write "robotPos"("initialPos") -> ()
      n4 = call "UDP_Receive_NEW_20170828.vi"("address"="234.5.6.7", "receiver port"=u16 55555) -> ("output array"=w3:bool[][], "roadblock names"=→"roadblock names":string[], "raw string data"=→"raw string data":string)  [unwired: 7 in]
      n5 = Or(x=bool[][] [[FALSE, FALSE, FALSE, FALSE, FALSE, FALSE, FALSE], [FALSE, TRUE, FALSE, TRUE, FALSE, TRUE, FALSE], [FALSE, FALSE, FALSE, FALSE, FALSE, FALSE, FALSE], [FALSE, TRUE, FALSE, TRUE, FALSE, TRUE, FALSE], [FALSE, FALSE, FALSE, FALSE, FALSE, FALSE, FALSE]] ("buildings"), y=w3) -> (x .or. y?=w2:bool[][])
    }
    frame #1 {
      # "Encoder Odometry"
      n6 = flat-sequence {
        frame #0 {
          n7 = while {
            stop <- w59 stop-if-true
            n8 = local read "stop"() -> (w61:bool)
            n9 = call "buttonTest.vi"() -> ("button"=w57:bool)  [unwired: 8 in, 3 out]
            n10 = Or(x=w61, y=w57) -> (x .or. y?=w60:bool)
            n11 = Or(x="go", y=w60) -> (x .or. y?=w59:bool)
            "speed" <- 0.0 ("speed")
          }
        }
        frame #1 {
          n12 = while {
            stop <- w68 stop-if-true
            n13 = Not(x="pause") -> (.not. x?=w63:bool)
            n14 = Boolean To (0,1)(Boolean=w63) -> (0, 1=w65:i16)
            n15 = Multiply(x="Max. Speed", y=w65) -> (x*y=w67:dbl)
            n16 = local write "speed"(w67) -> ()
            n17 = local read "stop"() -> (w68:bool)
          }
        }
      }
      n18 = flat-sequence {
        frame #0 {
          n19 = Wait Until Next ms Multiple(millisecond multiple=u32 500) -> ()  [unwired: 1 out]
        }
        frame #1 {
          n20 = local read "initialPos"() -> (w104:cluster{"xPos":dbl, "yPos":dbl, "Theta":dbl})
          n21 = Unbundle By Name(w104) -> ("xPos"=w103:dbl, "yPos"=w102:dbl)
          n22 = Build Array(w103) -> (w101:dbl[])
          n23 = Build Array(w102) -> (w100:dbl[])
          n24 = while {
            shift-right: [w126] -> _
            shift-left: w101 -> [w127]
            shift-right: [w125] -> _
            shift-left: w100 -> [w128]
            shift-right: [w111] -> _
            shift-left: w100 -> [w115]
            shift-right: [w110] -> _
            shift-left: w101 -> [w112]
            stop <- w109 stop-if-true
            n25 = Wait Until Next ms Multiple(millisecond multiple=u32 1) -> ()  [unwired: 1 out]
            n26 = local read "lidarRobotPos"() -> (w116:cluster{"xPos":dbl, "yPos":dbl, "Theta":dbl})
            n27 = local read "nextPoint"() -> (w123:cluster{"y":dbl, "x":dbl, "stop?":bool})
            n28 = local read "robotPos"() -> (w108:cluster{"xPos":dbl, "yPos":dbl, "Theta":dbl})
            n29 = Unbundle By Name(w108) -> ("xPos"=w107:dbl, "yPos"=w106:dbl)
            n30 = Unbundle By Name(w116) -> ("xPos"=w113:dbl, "yPos"=w114:dbl)
            n31 = Unbundle By Name(w123) -> ("y"=w120:dbl, "x"=w121:dbl)
            n32 = Insert Into Array(array=w127, new element=w107) -> (w126:dbl[])  [unwired: 1 in]
            n33 = Insert Into Array(array=w128, new element=w106) -> (w125:dbl[])  [unwired: 1 in]
            n34 = Insert Into Array(array=w112, new element=w113) -> (w110:dbl[])  [unwired: 1 in]
            n35 = Insert Into Array(array=w115, new element=w114) -> (w111:dbl[])  [unwired: 1 in]
            n36 = Build Array(w121) -> (w118:dbl[])
            n37 = Build Array(w120) -> (w119:dbl[])
            n38 = Bundle(w126, w125) -> (w124:cluster{dbl[], dbl[]})  [unwired: 1 in]
            n39 = Bundle(w118, w119) -> (w117:cluster{dbl[], dbl[]})  [unwired: 1 in]
            n40 = Bundle(w110, w111) -> (w105:cluster{dbl[], dbl[]})  [unwired: 1 in]
            n41 = call "Map.vi"() -> ("appended array"=w130:cluster{"Array":dbl[], "Array 2":dbl[]}[])  [unwired: 1 in]
            n42 = Insert Into Array(array=w130, new element #1=w124, new element #2=w117, new element #3=w105) -> (→"Field Map":cluster{"Array":dbl[], "Array 2":dbl[]}[])  [unwired: 1 in]
            n43 = local read "stop"() -> (w109:bool)
          }
        }
      }
      n44 = call "initialise.vi"() -> ("error out"=w15:errorcluster, "VISA resource name out"=w16:refnum<visa-resource-name>)  [unwired: 4 in]
      n45 = flat-sequence {
        tunnel: w11 -> [w22]
        frame #0 {
          # "Move to first Pickup Point"
          # "A-star for grid"
          n46 = Select(t="manualRoadblocks", s="USE MANUAL ROADBLOCKS", f=w22) -> (s? t:f=w21:bool[][])
          "path" <- w21
          n47 = call "waypoints.vi"("picupLocations"="pickupLocations", "roadBlocks"=w21) -> ("waypoints"=w25:cluster{"y":dbl, "x":dbl, "stop?":bool}[])  [unwired: 2 in]
          n48 = for {
            tunnel: w25 -> [w27] mode=indexing
            n49 = while {
              tunnel: w27 -> [w45]
              shift-right: [w40] -> _
              shift-left: cluster{"left":dbl, "right":dbl} {"left"=0.0, "right"=0.0} ("outputSpeed") -> [w41]
              stop <- w43 stop-if-true
              n50 = Tick Count (ms)() -> (millisecond timer value=w34:u32)
              n51 = local read "robotPos"() -> (w38:cluster{"xPos":dbl, "yPos":dbl, "Theta":dbl})
              n52 = Quotient & Remainder(x=w34, y=u32 5000) -> (x-y*floor(x/y)=w32:u32)  [unwired: 1 out]
              n53 = call "movement.vi"("nextPos"=w45, "robotPos"=w38) -> ("stop?"=w36:bool, "arrived?"=w37:bool, "outputSpeed"=w39:cluster{"left":dbl, "right":dbl})  [unwired: 1 in]
              n54 = Less?(x=w32, y=u32 1000) -> (x < y?=w30:bool)
              n55 = local read "stop"() -> (w44:bool)
              n56 = And(x=w37, y=w36) -> (x .and. y?=w35:bool)
              n57 = case shown="True" w35 {
                frame False {
                }
                frame True {
                  n58 = while {
                    stop <- w51 stop-if-true
                    n59 = local read "stop"() -> (w55:bool)
                    n60 = call "buttonTest.vi"() -> ("button"=w53:bool)  [unwired: 8 in, 3 out]
                    n61 = Or(x=w53, y=w55) -> (x .or. y?=w52:bool)
                    n62 = local read "go"() -> (w50:bool)
                    n63 = Or(x=w52, y=w50) -> (x .or. y?=w51:bool)
                    n64 = Wait (ms)(milliseconds to wait=u32 1) -> ()  [unwired: 1 out]
                  }
                }
              }
              n65 = local read "speed"() -> (w29:dbl)
              n66 = Or(x=w37, y=w44) -> (x .or. y?=w43:bool)
              n67 = case shown="False" w30 {
                tunnel: w29 -> [w46 _]
                tunnel: [w46 0.0 ("speed")] -> w28
                frame False {
                  w47 = u16 0 items=["Odometry", "Lidar"] ("Source")
                  n68 = local write "Source"(w47) -> ()
                }
                frame True {
                  w49 = u16 1 items=["Odometry", "Lidar"] ("Source")
                  n69 = local write "Source"(w49) -> ()
                }
              }
              n70 = Wait (ms)(milliseconds to wait=u32 2) -> ()  [unwired: 1 out]
              n71 = call "driveController.vi"("Max. Speed"=w28, "Stop?"=w43, "currentSpeed"=w41, "inputSpeed"=w39) -> ("outputSpeed"=w40:cluster{"left":dbl, "right":dbl})
              "nextPoint" <- w45
            }
          }
        }
        frame #1 {
          n72 = local write "stop"(TRUE ("stop")) -> ()
        }
      }
      n73 = local read "initialPos"() -> (w12:cluster{"xPos":dbl, "yPos":dbl, "Theta":dbl})
      n74 = while {
        tunnel: w16 -> [w98]
        tunnel: w15 -> [w97]
        tunnel: [w96] -> w14
        tunnel: [w95] -> w13
        stop <- w84 stop-if-true
        w77 = u16 1 items=["Shift to center", "Shift to lidar"] ("Shift type")
        w78 = u16 0 items=["Shift to center", "Shift to lidar"] ("Shift type")
        n75 = Wait (ms)(milliseconds to wait=u32 50) -> ()  [unwired: 1 out]
        n76 = local read "robotPos"() -> (w70:cluster{"xPos":dbl, "yPos":dbl, "Theta":dbl})
        n77 = call "lidarAdjust.vi"("Shift type"=w77, "input"=w70) -> ("shifted"=w72:cluster{"xPos":dbl, "yPos":dbl, "Theta":dbl})  [unwired: 1 in]
        n78 = call "readLidar.vi"("robotPos"=w72, "error in"=w97, "VISA resource name in"=w98) -> ("error out"=w95:errorcluster, "VISA resource name out"=w96:refnum<visa-resource-name>, "line out"=w71:cluster{"Line":cluster{"X":dbl, "Y":dbl}[]}[])  [unwired: 3 in, 1 out]
        n79 = Index Array(array=w71) -> (element=w93:cluster{"Line":cluster{"X":dbl, "Y":dbl}[]})  [unwired: 1 in]
        n80 = call "split.vi"("Threshold"="split theshold", "points in"=w93) -> ("line out"=w89:cluster{"Line":cluster{"X":dbl, "Y":dbl}[]}[])  [unwired: 9 in]
        n81 = call "lineFilter.vi"("min line size"="min line size", "Input"=w89) -> ("Output"=w88:cluster{"Line":cluster{"X":dbl, "Y":dbl}[]}[])  [unwired: 9 in]
        n82 = call "angleFilter.vi"("max angle deviation"="max angle deviation", "Input"=w88) -> ("Output"=w86:cluster{"Line":cluster{"X":dbl, "Y":dbl}[]}[])  [unwired: 9 in]
        n83 = call "merge.vi"("Merge Threshold"="merge threshold", "Input"=w86) -> ("Output"=w76:cluster{"Line":cluster{"X":dbl, "Y":dbl}[]}[])  [unwired: 9 in]
        n84 = call "lidarAngle.vi"("Input"=w76) -> ("average"=w75:dbl)  [unwired: 10 in]
        n85 = call "rotatePoints.vi"("robotPos"=w72, "angle shift"=w75, "Input"=w76) -> ("Output"=w73:cluster{"Line":cluster{"X":dbl, "Y":dbl}[]}[])  [unwired: 8 in]
        "rotated coordinate system" <- w73
        n86 = call "findCorners.vi"("robotPos"=w72, "Input"=w73) -> ("Output"=w74:cluster{"Line":cluster{"X":dbl, "Y":dbl}[]}[])  [unwired: 9 in]
        n87 = Index Array(array=w74, index=0) -> (element=w82:cluster{"Line":cluster{"X":dbl, "Y":dbl}[]})
        n88 = Unbundle(w82) -> ("Line"=w81:cluster{"X":dbl, "Y":dbl}[])
        n89 = call "lidarPos.vi"("robotPos"=w72, "angle deviation"=w75, "landmarks"="landmarks", "corners"=w81, "acceptance threshold"="point merge threshold") -> ("lidarPos"=w79:cluster{"xPos":dbl, "yPos":dbl, "theta":dbl})  [unwired: 6 in]
        n90 = call "lidarAdjust.vi"("Shift type"=w78, "input"=w79) -> ("shifted"=→"lidarRobotPos":cluster{"xPos":dbl, "yPos":dbl, "Theta":dbl})  [unwired: 1 in]
        n91 = local read "stop"() -> (w84:bool)
      }
      n92 = Bundle(0, 0) -> (w19:cluster{i32, i32})  [unwired: 1 in]
      n93 = while {
        shift-right: [w131] -> _
        shift-left: w12 -> [w142]
        shift-right: [w134] -> _
        shift-left: w19 -> [w133]
        i -> [w144]
        stop <- w138 stop-if-true
        n94 = Equal?(x=0, y=w144) -> (x = y?=w140:bool)
        n95 = call "encoderRead.vi"("previousEncoderCounts"=w133, "reset?"=w140) -> ("encoderCounts"=w134:cluster{"dRight":i32, "dLeft":i32}, "deltaEncoderCounts"=w132:cluster{"dRight":i32, "dLeft":i32})
        n96 = local read "lidarRobotPos"() -> (w137:cluster{"xPos":dbl, "yPos":dbl, "Theta":dbl})
        n97 = call "odomPos.vi"("encoderCounts"=w132, "posInput"=w142) -> ("posOutput"=w141:cluster{"xPos":dbl, "yPos":dbl, "Theta":dbl})  [unwired: 1 in]
        n98 = Wait Until Next ms Multiple(millisecond multiple=u32 1) -> ()  [unwired: 1 out]
        n99 = call "overwritePos.vi"("overwrite angle"="overwrite angle", "Source"="Source", "lidarPosInput"=w137, "odomPosInput"=w141) -> ("posOutput"=w131:cluster{"xPos":dbl, "yPos":dbl, "Theta":dbl})  [unwired: 1 in]
        "robotPos" <- w131
        n100 = local read "stop"() -> (w138:bool)
      }
      n101 = call "terminateLidar.vi"("error in"=w13, "VISA resource name"=w14) -> ()  [unwired: 3 in, 1 out]
    }
  }
